vi "Note Popup Setup.vi"(8 "error in (no error)":errorcluster, 9 "SR Number":i32, 10 "This VI in":refnum<vi>, 11 "String in":refnum<vi>) -> (0 "error out":errorcluster, 2 "This VI out":refnum<vi>, 3 "String out":refnum<vi>)   [LabVIEW 2018]
uses:
  <vilib>/Utility/miscctls.llb/LVPositionTypeDef.ctl
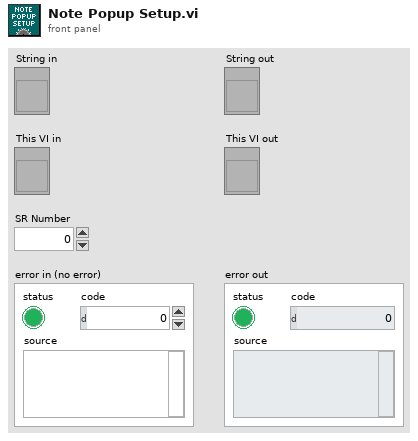
[diagram p1: front panel]
types:
  T1 = typedef "LVPositionTypeDef.ctl" = cluster{"Left":i32, "Top":i32}
  T2 = enum16{"Always On", "Always Off", "Off While Running"}
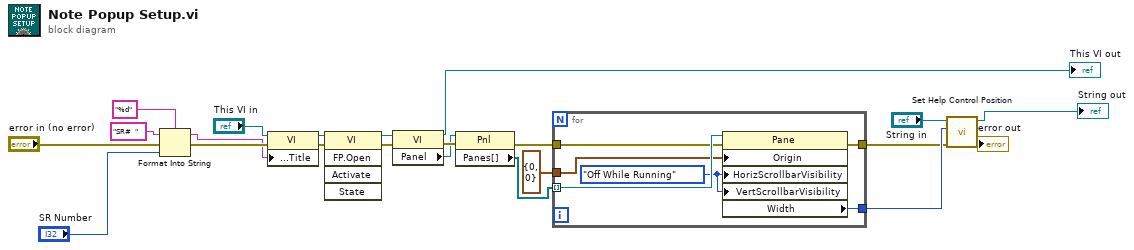
[diagram p0: block diagram]
diagram:
  n1 = Format Into String(format string="%d", initial string="SR#  ", error in="error in (no error)", "SR Number") -> (resulting string=w3:string, error out=w4:errorcluster)
  n2 = property class="VI"(reference="This VI in", error in=w4, "Front Panel.Title"=w3) -> (reference out=w16:refnum<vi>, error out=w17:errorcluster)
  n3 = invoke class="VI" method="FP.Open"(reference=w16, error in=w17) -> (reference out=w19:refnum<vi>, error out=w18:errorcluster)  [unwired: 3 in, 3 out]
  n4 = property class="VI"(reference=w19, error in=w18) -> (reference out=→"This VI out":refnum<vi>, error out=w21:errorcluster, "Panel"=w20:refnum<vi>)
  n5 = property class="Pnl"(reference=w20, error in=w21) -> (error out=w7:errorcluster, "Panes[]"=w8:refnum<vi>[])  [unwired: 1 out]
  n6 = for {
    tunnel: w8 -> [w28] mode=indexing
    tunnel: T1 {"Left"=0, "Top"=0} ("Position") -> [w27]
    tunnel: w7 -> [w26]
    tunnel: [w25] -> w10
    tunnel: [w23] -> w11
    w24 = T2."Off While Running" ("Horizontal Scrollbar Visibility")
    n7 = property class="Pane"(reference=w28, error in=w26, "Origin"=w27, "HorizScrollbarVisibility"=w24, "VertScrollbarVisibility"=w24) -> (error out=w25:errorcluster, "Width"=w23:u32)  [unwired: 1 out]
  }
  n8 = call "Set Help Control Position.vi"("error in (no error)"=w10, "Width"=w11, "String in"="String in") -> ("error out"=→"error out":errorcluster, "String out"=→"String out":refnum<vi>)  [unwired: 7 in]
